vi "Complicated Function Generator.vi"(0 "frequency":dbl=10.0 format="%0.2p", 1 "signal type":T2(ring), 3 "offset":dbl format="%0.2p", 5 "amplitude":dbl=4.0 format="%0.2p", 7 "samples":dbl=1000.0 format="%0.2p", 9 "bufsize":dbl=1000.0 format="%#.2p", 11 "error in (no error)":errorcluster, 12 "Chans":u32, 14 "Tab Control":T1(ring)) -> (4 "Wave out":waveform(dbl), 6 "WfmArray":waveform(dbl)[](array[waveform]), 8 "DblArray":dbl[][](array[numeric]), 10 "DBL Out":dbl[](array[numeric]), 13 "Sync":bool, 15 "error out":errorcluster)   [LabVIEW 2010]
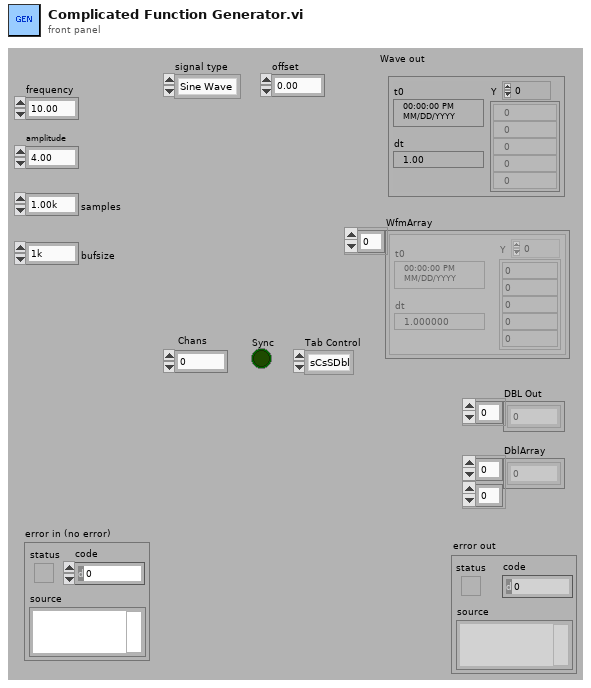
[diagram p1: front panel]
types:
  T1 = enum32{"sCsSDbl", "sCsSWfm", "sCnS1D", "sCnSWfm", "nCsSDbl", "nCsSWfm", "nCnS2D", "nCnS1DWfm", "2DI16", "2DI32", "2DU16", "2DU32"}
  T2 = enum16{"Sine Wave", "Triangle Wave", "Square Wave", "Sawtooth Wave"}
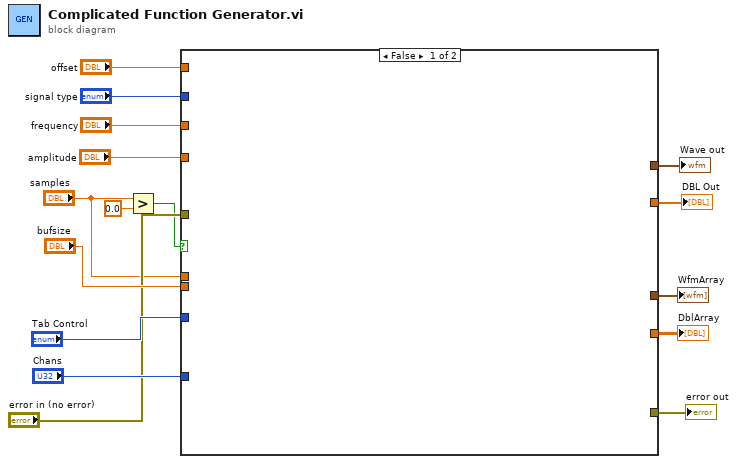
[diagram p0: block diagram]
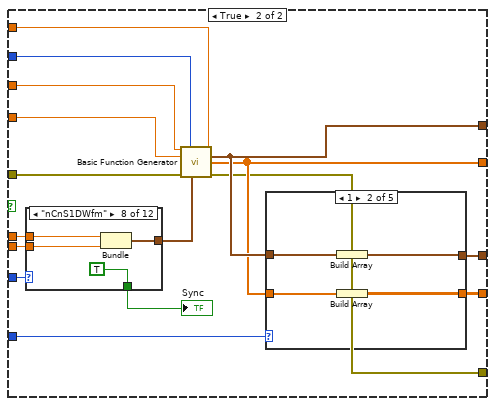
[diagram p2: hidden frame]
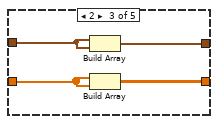
[diagram p4: hidden frame]
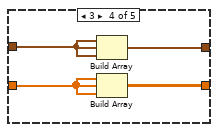
[diagram p5: hidden frame]
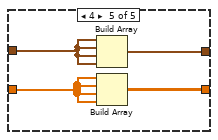
[diagram p6: hidden frame]
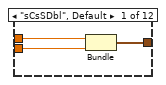
[diagram p7: hidden frame]
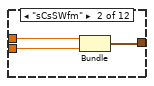
[diagram p8: hidden frame]
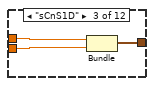
[diagram p9: hidden frame]
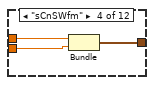
[diagram p10: hidden frame]
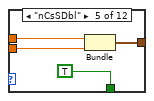
[diagram p11: hidden frame]
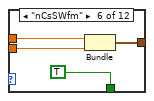
[diagram p12: hidden frame]
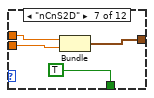
[diagram p13: hidden frame]
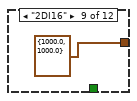
[diagram p14: hidden frame]
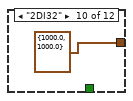
[diagram p15: hidden frame]
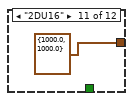
[diagram p16: hidden frame]
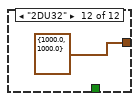
[diagram p17: hidden frame]
diagram:
  n1 = Greater?(x="samples", y=0.0) -> (0:w1:bool)
  n2 = case shown="False" w1 {
    tunnel: "signal type" -> [_ w32]
    tunnel: "frequency" -> [_ w31]
    tunnel: "amplitude" -> [_ w30]
    tunnel: "offset" -> [_ w28]
    tunnel: "samples" -> [_ w27]
    tunnel: "bufsize" -> [_ w26]
    tunnel: "Chans" -> [_ w25]
    tunnel: [_ w24] -> w10
    tunnel: [_ w23] -> w9
    tunnel: [_ w22] -> w8
    tunnel: [_ w21] -> w7
    tunnel: "Tab Control" -> [_ w20]
    tunnel: [_ w19] -> w5
    tunnel: "error in (no error)" -> [_ w18]
    frame False {
    }
    frame True {
      n3 = case shown="\"nCnS1DWfm\"" w20 {
        tunnel: [w49 w52 w57 w59 w64 w68 w70 w74 cluster{"samples":dbl, "bufsize":dbl} {"samples"=1000.0, "bufsize"=1000.0} cluster{"samples":dbl, "bufsize":dbl} {"samples"=1000.0, "bufsize"=1000.0} cluster{"samples":dbl, "bufsize":dbl} {"samples"=1000.0, "bufsize"=1000.0} cluster{"samples":dbl, "bufsize":dbl} {"samples"=1000.0, "bufsize"=1000.0}] -> w29
        tunnel: w27 -> [w51 w54 w56 w60 w63 w67 w72 w76 _ _ _ _]
        tunnel: w26 -> [w50 w53 w55 w58 w62 w66 w71 w75 _ _ _ _]
        tunnel: [_ _ _ _ TRUE TRUE TRUE TRUE _ _ _ _] -> w17
        frame "sCsSDbl", Default {
          n4 = Bundle("samples"=w51, "bufsize"=w50) -> (w49:cluster{"samples":dbl, "bufsize":dbl})  [unwired: 1 in]
        }
        frame "sCsSWfm" {
          n5 = Bundle("samples"=w54, "bufsize"=w53) -> (w52:cluster{"samples":dbl, "bufsize":dbl})  [unwired: 1 in]
        }
        frame "sCnS1D" {
          n6 = Bundle("samples"=w56, "bufsize"=w55) -> (w57:cluster{"samples":dbl, "bufsize":dbl})  [unwired: 1 in]
        }
        frame "sCnSWfm" {
          n7 = Bundle("samples"=w60, "bufsize"=w58) -> (w59:cluster{"samples":dbl, "bufsize":dbl})  [unwired: 1 in]
        }
        frame "nCsSDbl" {
          n8 = Bundle("samples"=w63, "bufsize"=w62) -> (w64:cluster{"samples":dbl, "bufsize":dbl})  [unwired: 1 in]
        }
        frame "nCsSWfm" {
          n9 = Bundle("samples"=w67, "bufsize"=w66) -> (w68:cluster{"samples":dbl, "bufsize":dbl})  [unwired: 1 in]
        }
        frame "nCnS2D" {
          n10 = Bundle("samples"=w72, "bufsize"=w71) -> (w70:cluster{"samples":dbl, "bufsize":dbl})  [unwired: 1 in]
        }
        frame "nCnS1DWfm" {
          n11 = Bundle("samples"=w76, "bufsize"=w75) -> (w74:cluster{"samples":dbl, "bufsize":dbl})  [unwired: 1 in]
        }
        frame "2DI16" {
        }
        frame "2DI32" {
        }
        frame "2DU16" {
        }
        frame "2DU32" {
        }
      }
      "Sync" <- w17
      n12 = call "Basic Function Generator.vi"("frequency"=w31, "signal type"=w32, "offset"=w28, "amplitude"=w30, "error in (no error)"=w18, "sampling info"=w29) -> ("signal out"=w24:waveform(dbl), "DBL Out"=w23:dbl[], "error out"=w19:errorcluster)  [unwired: 6 in, 1 out]
      n13 = case shown="1" w25 {
        tunnel: w24 -> [_ w36 w40 w44 w46]
        tunnel: [_ w35 w38 w41 w47] -> w22
        tunnel: w23 -> [_ w34 w39 w43 w45]
        tunnel: [_ w33 w37 w42 w48] -> w21
        frame 0, Default {
        }
        frame 1 {
          n14 = Build Array(w36) -> (w35:waveform(dbl)[])
          n15 = Build Array(w34) -> (w33:dbl[][])
        }
        frame 2 {
          n16 = Build Array(w40, w40) -> (w38:waveform(dbl)[])
          n17 = Build Array(w39, w39) -> (w37:dbl[][])
        }
        frame 3 {
          n18 = Build Array(w44, w44, w44) -> (w41:waveform(dbl)[])
          n19 = Build Array(w43, w43, w43) -> (w42:dbl[][])
        }
        frame 4 {
          n20 = Build Array(w46, w46, w46, w46) -> (w47:waveform(dbl)[])
          n21 = Build Array(w45, w45, w45, w45) -> (w48:dbl[][])
        }
      }
    }
  }
  "Wave out" <- w10
  "DBL Out" <- w9
  "WfmArray" <- w8
  "DblArray" <- w7
  "error out" <- w5
